vi "SR400.vi"(8 "error in (no error)":errorcluster, 10 "Settings In":T1={"Channel A"={"Input"=0, "A Discriminator Level (V)"=0.0, "A Discriminator Slope"=enum."Falling", "A Gate Mode"=enum."CW", "A Gate Delay (s)"=0.0, "A Gate Width (s)"=5e-09, "Scan Increment (s)"=0.0}, "Channel B"={"Input"=0, "B Discriminator Level (V)"=0.0, "B Discriminator Slope"=enum."Falling", "B Gate Mode"=enum."CW", "B Gate Delay (s)"=0.0, "B Gate Width (s)"=5e-09, "Scan Increment (s)"=0.0}, "Channel T"={"Input"=0, "Trigger Level (V)"=0.0, "Trigger Slope"=enum."Falling", "T Discriminator Slope"=enum."Falling", "T Discriminator Level (V)"=0.0, "Trigger Preset"=1.0}, "N Periods"=0.0, "At N"=enum."Stop", "Counting Mode"=enum."A,B for T Preset", "GPIB Address"="", "Dwell Time (s)"=0.002, "Port 1 Mode"=0, "Port 1 Voltage"=0.0, "Port 1 Scan Increment"=-0.5, "Port 2 Voltage"=0.0, "Port 2 Scan Increment"=0.0, "Port 2 Mode"=0, "Counter Toggle"=FALSE, "Pusleblater Settings"={"Loop Start Channel"=0.0, "Loop End Channel"=0.0, "Loop On"=FALSE}} {"Port 2 Mode" items=["Scan"=1, "Fixed"=0]; "Port 2 Scan Increment" min=-0.5 max=0.5; "Port 2 Voltage" min=-10.0 max=10.0; "Port 1 Scan Increment" min=-0.5 max=-0.5; "Port 1 Voltage" min=-10.0 max=10.0; "Port 1 Mode" items=["Scan"=1, "Fixed"=0]; "Dwell Time (s)" min=0.002 max=60.0 format="%#_6p"; "N Periods" min=0.0 max=2000.0 step=1.0; "Channel T"."Trigger Preset" min=1.0 max=900000000000.0 format="%#_1e"; "Channel T"."T Discriminator Level (V)" min=-0.3 max=0.3 format="%#_6p"; "Channel T"."Trigger Level (V)" min=-2.0 max=2.0 format="%#_6p"; "Channel T"."Input" items=["10 MHz", "Input 2", "Trig"]; "Channel B"."Scan Increment (s)" min=0.0 max=0.09992 format="%#_6p"; "Channel B"."B Gate Width (s)" min=5e-09 max=0.9992 format="%#_6p"; "Channel B"."B Gate Delay (s)" min=0.0 max=0.9992 format="%#_6p"; "Channel B"."B Discriminator Level (V)" min=-0.3 max=0.3 format="%#_6p"; "Channel B"."Input" items=["Input 2"=2, "Input 1"=1]; "Channel A"."Scan Increment (s)" min=0.0 max=0.09992 format="%#_6p"; "Channel A"."A Gate Width (s)" min=5e-09 max=0.9992 format="%#_6p"; "Channel A"."A Gate Delay (s)" min=0.0 max=0.9992 format="%#_6p"; "Channel A"."A Discriminator Level (V)" min=-0.3 max=0.3 format="%#_6p"; "Channel A"."Input" items=["Input 1", "10 MHz"]}) -> (0 "error out":errorcluster, 2 "Settings Out":T1={"Channel A"={"Input"=0, "A Discriminator Level (V)"=0.0, "A Discriminator Slope"=enum."Falling", "A Gate Mode"=enum."CW", "A Gate Delay (s)"=0.0, "A Gate Width (s)"=5e-09, "Scan Increment (s)"=0.0}, "Channel B"={"Input"=0, "B Discriminator Level (V)"=0.0, "B Discriminator Slope"=enum."Falling", "B Gate Mode"=enum."CW", "B Gate Delay (s)"=0.0, "B Gate Width (s)"=5e-09, "Scan Increment (s)"=0.0}, "Channel T"={"Input"=0, "Trigger Level (V)"=0.0, "Trigger Slope"=enum."Falling", "T Discriminator Slope"=enum."Falling", "T Discriminator Level (V)"=0.0, "Trigger Preset"=1.0}, "N Periods"=0.0, "At N"=enum."Stop", "Counting Mode"=enum."A,B for T Preset", "GPIB Address"="", "Dwell Time (s)"=0.002, "Port 1 Mode"=0, "Port 1 Voltage"=0.0, "Port 1 Scan Increment"=-0.5, "Port 2 Voltage"=0.0, "Port 2 Scan Increment"=0.0, "Port 2 Mode"=0, "Counter Toggle"=FALSE, "Pusleblater Settings"={"Loop Start Channel"=0.0, "Loop End Channel"=0.0, "Loop On"=FALSE}} {"Port 2 Mode" items=["Scan"=1, "Fixed"=0]; "Port 2 Scan Increment" min=-0.5 max=0.5; "Port 2 Voltage" min=-10.0 max=10.0; "Port 1 Scan Increment" min=-0.5 max=-0.5; "Port 1 Voltage" min=-10.0 max=10.0; "Port 1 Mode" items=["Scan"=1, "Fixed"=0]; "Dwell Time (s)" min=0.002 max=60.0 format="%#_6p"; "N Periods" min=0.0 max=2000.0 step=1.0; "Channel T"."Trigger Preset" min=1.0 max=900000000000.0 format="%#_1e"; "Channel T"."T Discriminator Level (V)" min=-0.3 max=0.3 format="%#_6p"; "Channel T"."Trigger Level (V)" min=-2.0 max=2.0 format="%#_6p"; "Channel T"."Input" items=["10 MHz", "Input 2", "Trig"]; "Channel B"."Scan Increment (s)" min=0.0 max=0.09992 format="%#_6p"; "Channel B"."B Gate Width (s)" min=5e-09 max=0.9992 format="%#_6p"; "Channel B"."B Gate Delay (s)" min=0.0 max=0.9992 format="%#_6p"; "Channel B"."B Discriminator Level (V)" min=-0.3 max=0.3 format="%#_6p"; "Channel B"."Input" items=["Input 2"=2, "Input 1"=1]; "Channel A"."Scan Increment (s)" min=0.0 max=0.09992 format="%#_6p"; "Channel A"."A Gate Width (s)" min=5e-09 max=0.9992 format="%#_6p"; "Channel A"."A Gate Delay (s)" min=0.0 max=0.9992 format="%#_6p"; "Channel A"."A Discriminator Level (V)" min=-0.3 max=0.3 format="%#_6p"; "Channel A"."Input" items=["Input 1", "10 MHz"]})   [LabVIEW 2015]
uses:
  Controls/SR400/SR400.ctl
  Controls/SR400/Channel A/channelA.ctl
  Controls/SR400/Channel A/channelA_inputs.ctl
  Controls/SR400/discrim_slope.ctl
  Controls/SR400/gate_mode.ctl
  Controls/SR400/Channel B/channelB.ctl
  Controls/SR400/Channel B/inputsB.ctl
  Controls/SR400/Channel T/channelT.ctl
  Controls/SR400/Channel T/inputsT.ctl
  <vilib>/Instr/_visa.llb/GPIB Status Boolean Array.ctl
  Controls/SR400/sr400_states.ctl
panel:
  out "Port command":string caption="Result"
  out "Status after writing ports":T10
  out "Scan command":string caption="Result"
  out "Status after writing scan":T10
  out "Counter T Command":string caption="Result"
  out "Status after writing T":T10
  out "Counter B Command":string caption="Result"
  out "Status after writing B":T10
  out "Status after writing A":T10
  out "Counter A Command":string caption="Result"
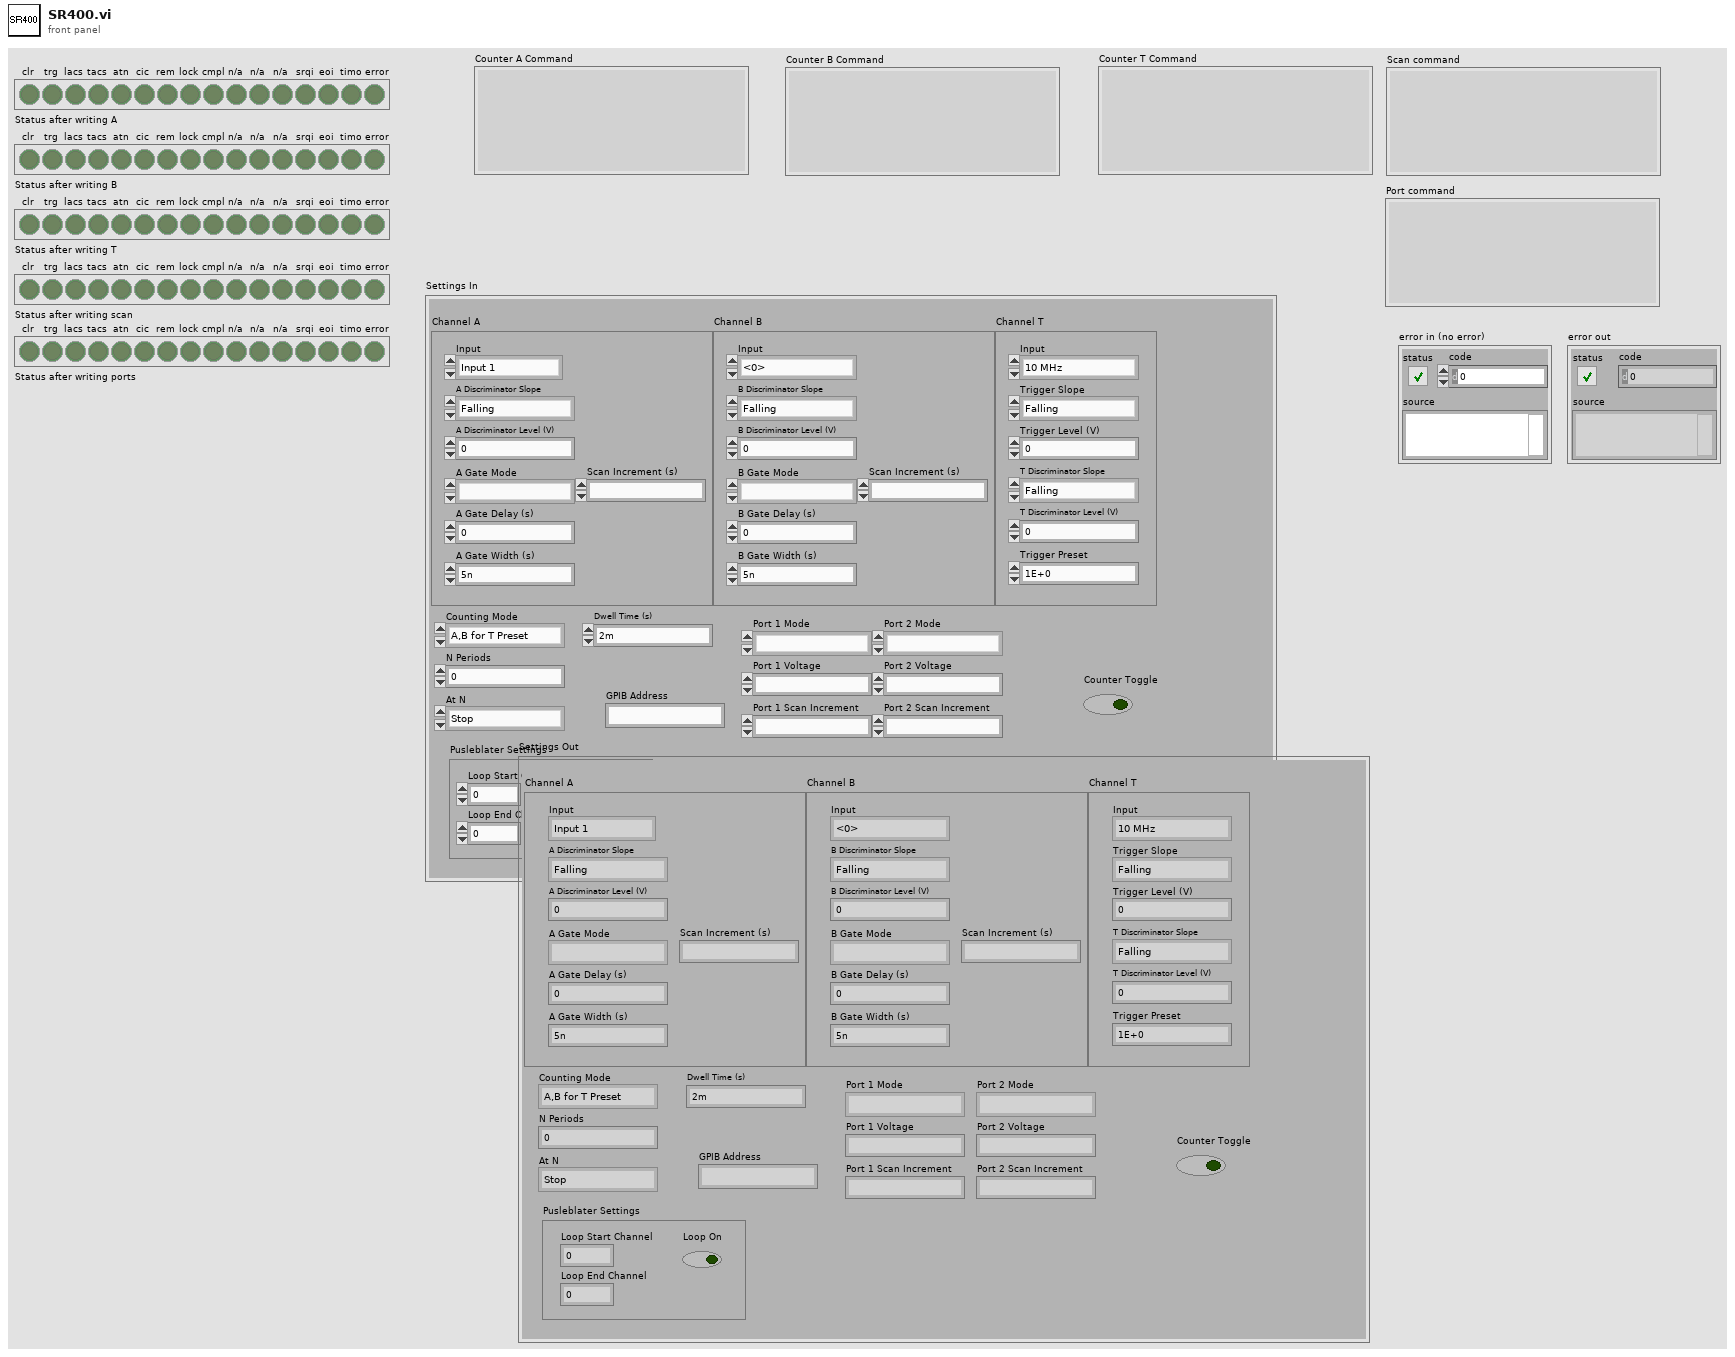
[diagram p1: front panel]
types:
  T1 = typedef "SR400.ctl" = cluster{"Channel A":T2, "Channel B":T6, "Channel T":T8, "N Periods":dbl, "At N":enum16{"Stop", "Start"}, "Counting Mode":enum16{"A,B for T Preset", "A-B for T Preset", "A+B for T Preset"}, "GPIB Address":string, "Dwell Time (s)":dbl, "Port 1 Mode":i32, "Port 1 Voltage":dbl, "Port 1 Scan Increment":dbl, "Port 2 Voltage":dbl, "Port 2 Scan Increment":dbl, "Port 2 Mode":i32, "Counter Toggle":bool, "Pusleblater Settings":cluster{"Loop Start Channel":dbl, "Loop End Channel":dbl, "Loop On":bool}}
  T2 = typedef "channelA.ctl" = cluster{"Input":T3, "A Discriminator Level (V)":dbl, "A Discriminator Slope":T4, "A Gate Mode":T5, "A Gate Delay (s)":dbl, "A Gate Width (s)":dbl, "Scan Increment (s)":dbl}
  T3 = typedef "channelA_inputs.ctl" = u16
  T4 = typedef "discrim_slope.ctl" = enum16{"Rising", "Falling"}
  T5 = typedef "gate_mode.ctl" = enum16{"CW", "Fixed", "Scan"}
  T6 = typedef "channelB.ctl" = cluster{"Input":T7, "B Discriminator Level (V)":dbl, "B Discriminator Slope":T4, "B Gate Mode":T5, "B Gate Delay (s)":dbl, "B Gate Width (s)":dbl, "Scan Increment (s)":dbl}
  T7 = typedef "inputsB.ctl" = u16
  T8 = typedef "channelT.ctl" = cluster{"Input":T9, "Trigger Level (V)":dbl, "Trigger Slope":T4, "T Discriminator Slope":T4, "T Discriminator Level (V)":dbl, "Trigger Preset":dbl}
  T9 = typedef "inputsT.ctl" = u16
  T10 = typedef "GPIB Status Boolean Array.ctl" = bool[]
  T11 = typedef "sr400_states.ctl" = enum16{"Check Toggle", "Initialize", "Write A Settings", "Write B Settings", "Write T Settings", "Write Scan Settings", "Write Port Settings", "End"}
  T12 = enum16{"A,B for T Preset", "A-B for T Preset", "A+B for T Preset"}
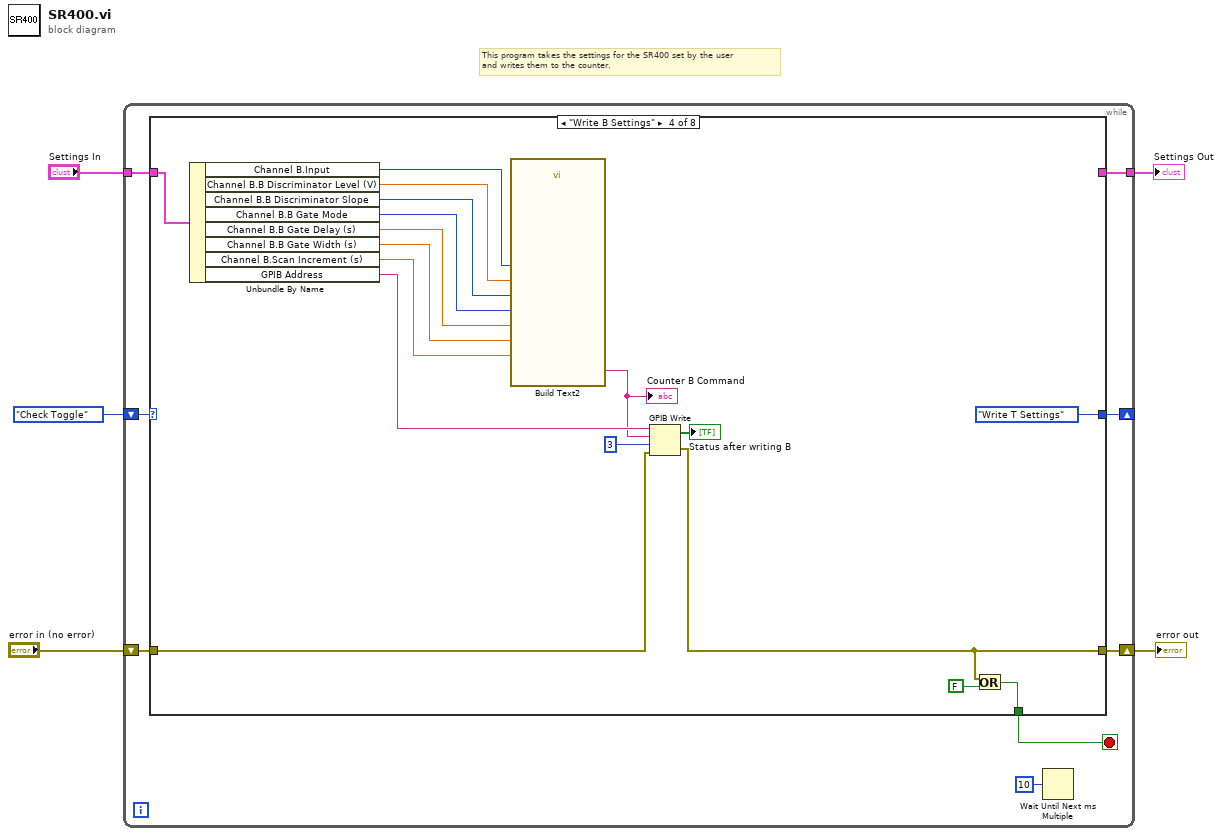
[diagram p0: block diagram]
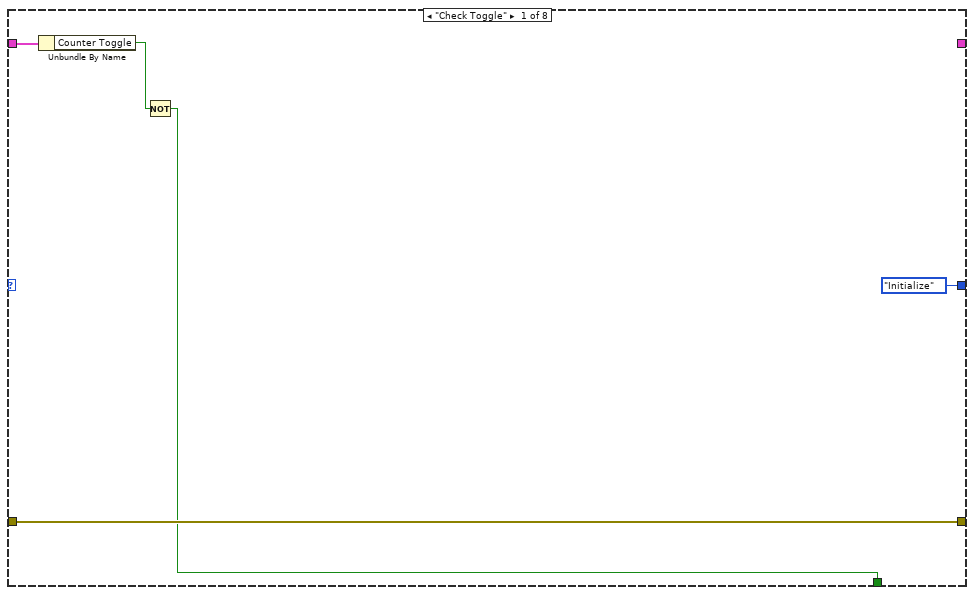
[diagram p2: hidden frame]
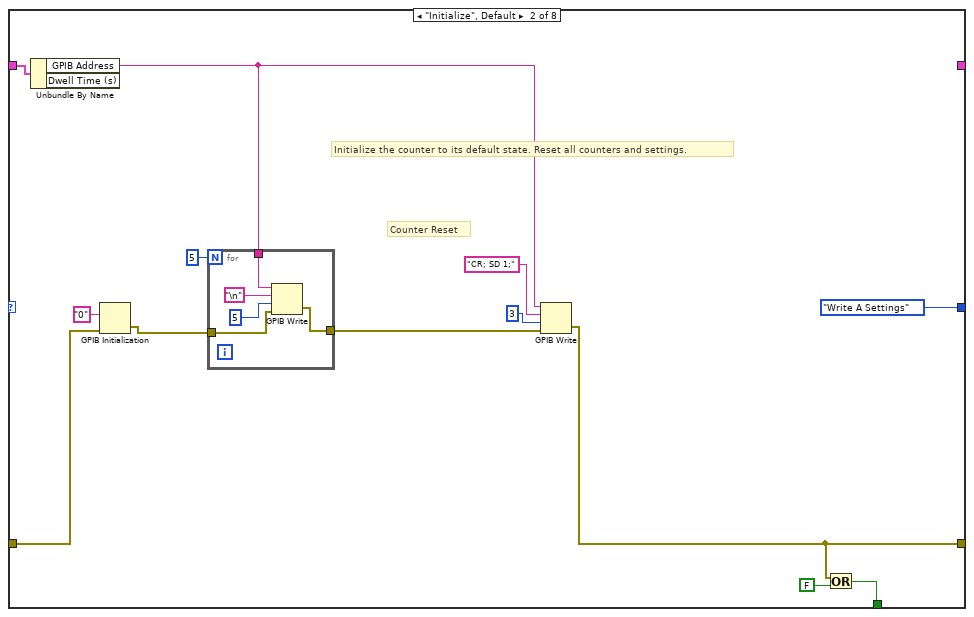
[diagram p3: hidden frame]
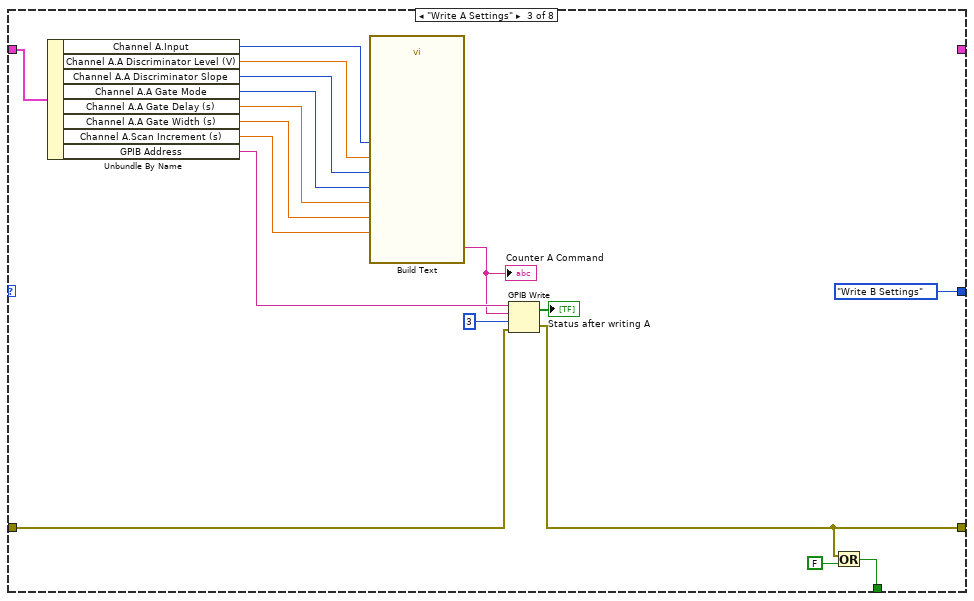
[diagram p4: hidden frame]
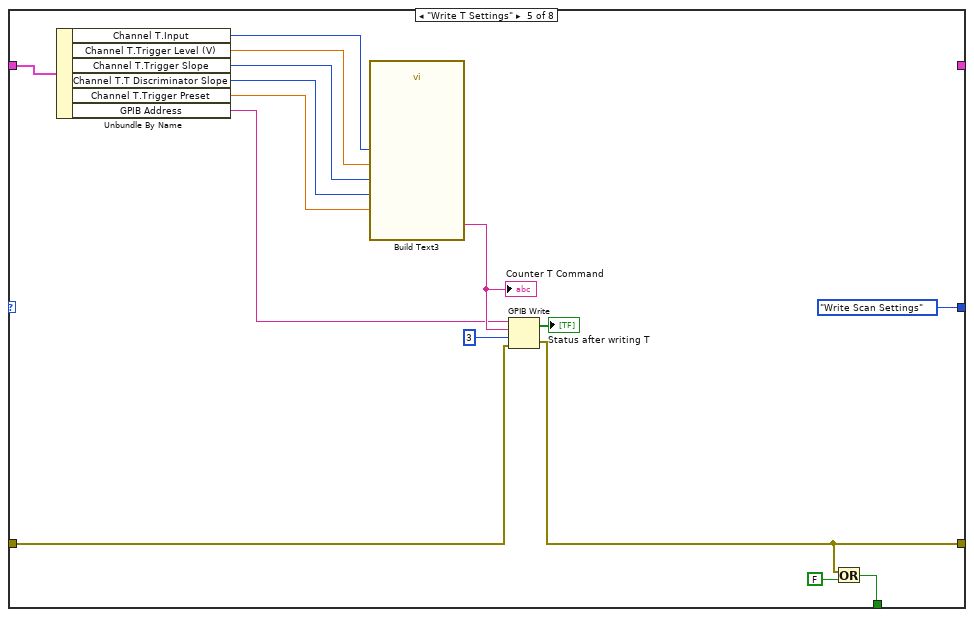
[diagram p5: hidden frame]
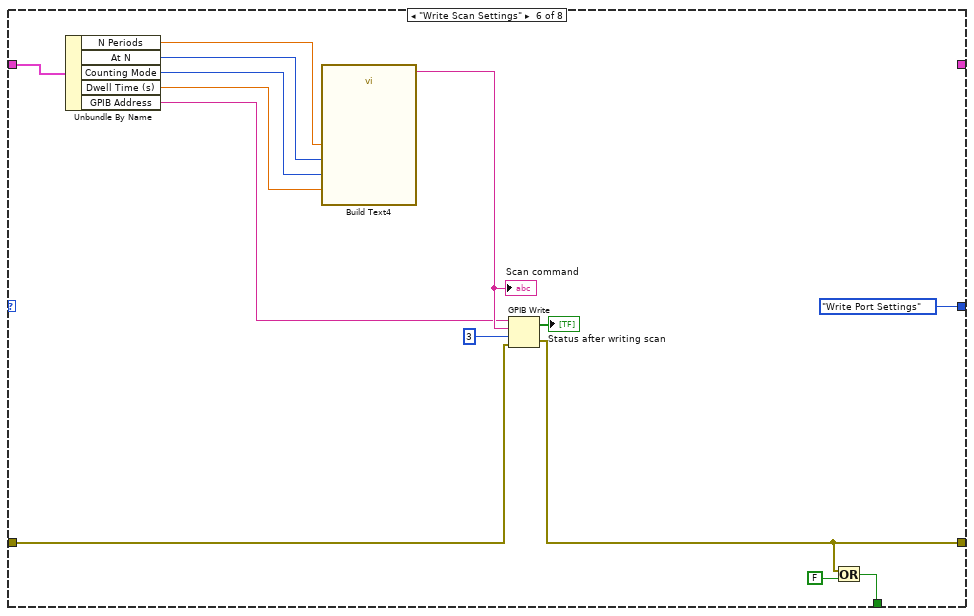
[diagram p6: hidden frame]
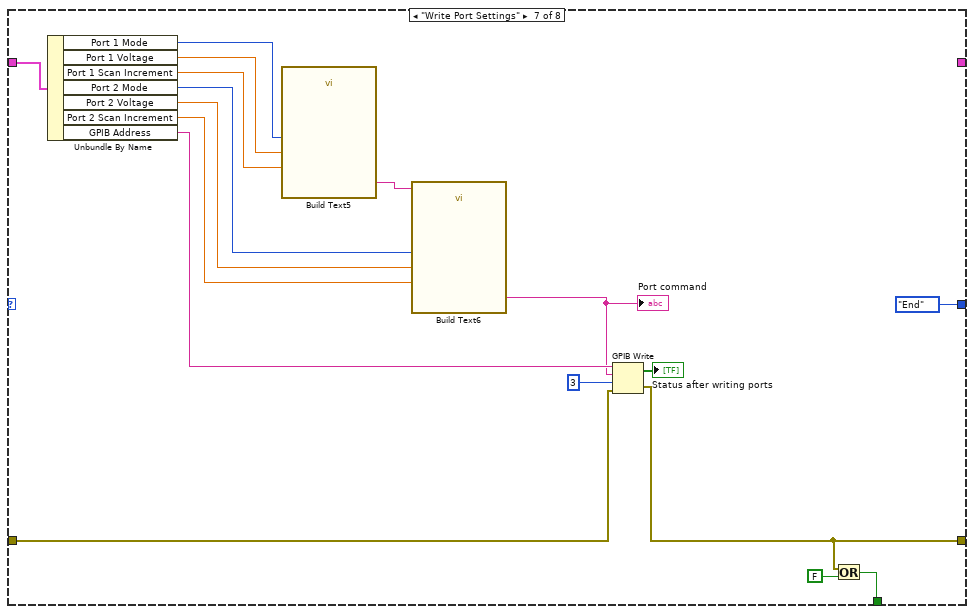
[diagram p7: hidden frame]
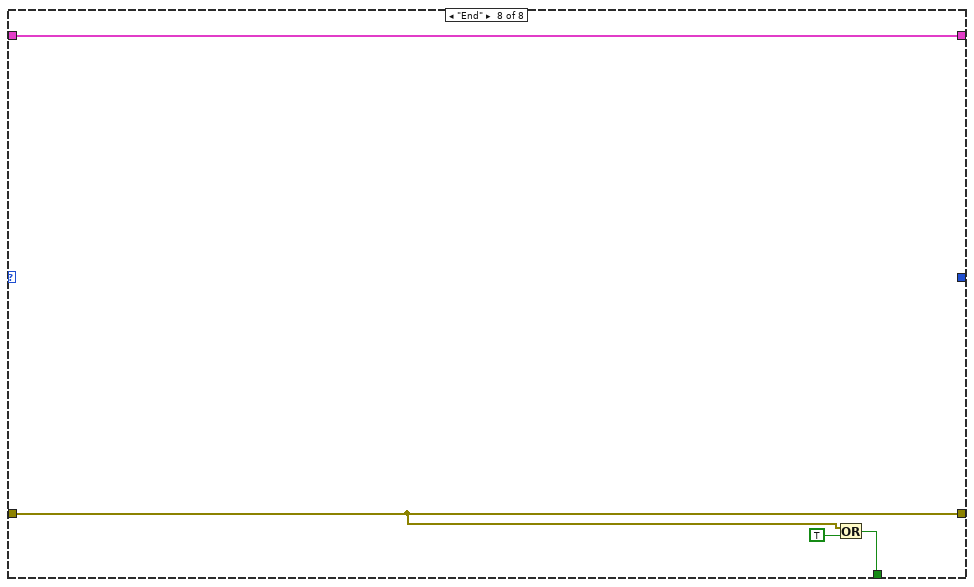
[diagram p8: hidden frame]
diagram:
  # "This program takes the settings for the SR400 set by the user\nand writes them to the counter."
  n1 = while {
    shift-right: [w11] -> _
    shift-left: sr400_states."Check Toggle" -> [w13]
    tunnel: "Settings In" -> [w10]
    shift-right: [w9] -> w2
    shift-left: "error in (no error)" -> [w12]
    tunnel: [w7] -> w1
    stop <- w8 stop-if-true
    n2 = case shown="\"Write B Settings\"" w13 {
      tunnel: w12 -> [w18 w27 w43 w60 w79 w94 w111 w118]
      tunnel: [sr400_states."Initialize" sr400_states."Write A Settings" sr400_states."Write B Settings" sr400_states."Write T Settings" sr400_states."Write Scan Settings" sr400_states."Write Port Settings" sr400_states."End" _] -> w11
      tunnel: w10 -> [w17 w30 w53 w70 w85 w99 w116 w117]
      tunnel: [w18 w26 w40 w57 w76 w91 w108 w118] -> w9
      tunnel: [w14 w28 w42 w59 w78 w93 w110 w119] -> w8
      tunnel: [_ _ _ _ _ _ _ w117] -> w7
      frame "Check Toggle" {
        n3 = Unbundle By Name(w17) -> ("Counter Toggle"=w15:bool)
        n4 = Not(x=w15) -> (.not. x?=w14:bool)
      }
      frame "Initialize", Default {
        # "Counter Reset"
        # "Initialize the counter to its default state. Reset all counters and settings."
        n5 = Unbundle By Name(w30) -> ("GPIB Address"=w19:string)  [unwired: 1 out]
        n6 = GPIB Initialization(4:w27, 6:"0" ("address string")) -> (0:w21:errorcluster)  [unwired: 5 in]
        n7 = for {
          N: 5 -> [_]
          tunnel: w19 -> [w34]
          tunnel: w21 -> [w33]
          tunnel: [w32] -> w20
          n8 = GPIB Write(0:w34, 1:"\n", 2:5 ("timeout ms (488.2 global)"), 3:w33) -> (6:w32:errorcluster)  [unwired: 1 in, 1 out]
        }
        n9 = GPIB Write(0:w19, 1:"CR; SD 1;" ("data"), 2:i16 3 ("mode (0)"), 3:w20) -> (6:w26:errorcluster)  [unwired: 1 in, 1 out]
        n10 = Or(x=w26, y=FALSE) -> (x .or. y?=w28:bool)
      }
      frame "Write A Settings" {
        n11 = Unbundle By Name(w53) -> ("Channel A.Input"=w52:T3, "Channel A.A Discriminator Level (V)"=w51:dbl, "Channel A.A Discriminator Slope"=w50:T4, "Channel A.A Gate Mode"=w49:T5, "Channel A.A Gate Delay (s)"=w48:dbl, "Channel A.A Gate Width (s)"=w47:dbl, "Channel A.Scan Increment (s)"=w46:dbl, "GPIB Address"=w45:string)
        n12 = call "Build Text"("Gmode"=w49, "gwidth"=w47, "input"=w52, "Dlevel"=w51, "Dslope"=w50, "gdelay"=w48, "gstep"=w46) -> ("Result"=w37:string)  [unwired: 7 in, 1 out]
        "Counter A Command" <- w37
        n13 = GPIB Write(0:w45, 1:w37, 2:i16 3 ("mode (0)"), 3:w43) -> (5:→"Status after writing A":bool[], 6:w40:errorcluster)  [unwired: 1 in]
        n14 = Or(x=w40, y=FALSE) -> (x .or. y?=w42:bool)
      }
      frame "Write B Settings" {
        n15 = Unbundle By Name(w70) -> ("Channel B.Input"=w69:T7, "Channel B.B Discriminator Level (V)"=w68:dbl, "Channel B.B Discriminator Slope"=w67:T4, "Channel B.B Gate Mode"=w66:T5, "Channel B.B Gate Delay (s)"=w65:dbl, "Channel B.B Gate Width (s)"=w64:dbl, "Channel B.Scan Increment (s)"=w63:dbl, "GPIB Address"=w62:string)
        n16 = call "Build Text2"("Gmode"=w66, "gwidth"=w64, "input"=w69, "Dlevel"=w68, "Dslope"=w67, "gdelay"=w65, "gstep"=w63) -> ("Result"=w54:string)  [unwired: 7 in, 1 out]
        "Counter B Command" <- w54
        n17 = GPIB Write(0:w62, 1:w54, 2:i16 3 ("mode (0)"), 3:w60) -> (5:→"Status after writing B":bool[], 6:w57:errorcluster)  [unwired: 1 in]
        n18 = Or(x=w57, y=FALSE) -> (x .or. y?=w59:bool)
      }
      frame "Write T Settings" {
        n19 = Unbundle By Name(w85) -> ("Channel T.Input"=w84:T9, "Channel T.Trigger Level (V)"=w83:dbl, "Channel T.Trigger Slope"=w82:T4, "Channel T.T Discriminator Slope"=w81:T4, "Channel T.Trigger Preset"=w71:dbl, "GPIB Address"=w72:string)
        n20 = call "Build Text3"("TDslope"=w81, "input"=w84, "Tlevel"=w83, "Tslope"=w82, "tset"=w71) -> ("Result"=w73:string)  [unwired: 9 in, 1 out]
        "Counter T Command" <- w73
        n21 = GPIB Write(0:w72, 1:w73, 2:i16 3 ("mode (0)"), 3:w79) -> (5:→"Status after writing T":bool[], 6:w76:errorcluster)  [unwired: 1 in]
        n22 = Or(x=w76, y=FALSE) -> (x .or. y?=w78:bool)
      }
      frame "Write Scan Settings" {
        n23 = Unbundle By Name(w99) -> ("N Periods"=w98:dbl, "At N"=w97:enum16{"Stop", "Start"}, "Counting Mode"=w96:T12, "Dwell Time (s)"=w86:dbl, "GPIB Address"=w87:string)
        n24 = call "Build Text4"("dwell"=w86, "periods"=w98, "endscan"=w97, "countmode"=w96) -> ("Result"=w88:string)  [unwired: 10 in, 1 out]
        "Scan command" <- w88
        n25 = GPIB Write(0:w87, 1:w88, 2:i16 3 ("mode (0)"), 3:w94) -> (5:→"Status after writing scan":bool[], 6:w91:errorcluster)  [unwired: 1 in]
        n26 = Or(x=w91, y=FALSE) -> (x .or. y?=w93:bool)
      }
      frame "Write Port Settings" {
        n27 = Unbundle By Name(w116) -> ("Port 1 Mode"=w115:i32, "Port 1 Voltage"=w114:dbl, "Port 1 Scan Increment"=w113:dbl, "Port 2 Mode"=w104:i32, "Port 2 Voltage"=w103:dbl, "Port 2 Scan Increment"=w102:dbl, "GPIB Address"=w105:string)
        n28 = call "Build Text5"("pmode"=w115, "plevel"=w114, "pstep"=w113) -> ("Result"=w101:string)  [unwired: 11 in, 1 out]
        n29 = call "Build Text6"("Beginning Text"=w101, "pmode"=w104, "plevel"=w103, "pstep"=w102) -> ("Result"=w100:string)  [unwired: 10 in, 1 out]
        "Port command" <- w100
        n30 = GPIB Write(0:w105, 1:w100, 2:i16 3 ("mode (0)"), 3:w111) -> (5:→"Status after writing ports":bool[], 6:w108:errorcluster)  [unwired: 1 in]
        n31 = Or(x=w108, y=FALSE) -> (x .or. y?=w110:bool)
      }
      frame "End" {
        n32 = Or(x=w118, y=TRUE) -> (x .or. y?=w119:bool)
      }
    }
    n33 = Wait Until Next ms Multiple(millisecond multiple=u32 10) -> ()  [unwired: 1 out]
  }
  "error out" <- w2
  "Settings Out" <- w1
